vi "CoboltLaser_ComPortClose.vi"(0 "ComPort":refnum<visa-resource-name>, 5 "error in (no error)":errorcluster) -> (19 "error out":errorcluster)   [LabVIEW 2012, in "Cobolt.lvclass"]
uses:
  Template/Cobolt.lvclass
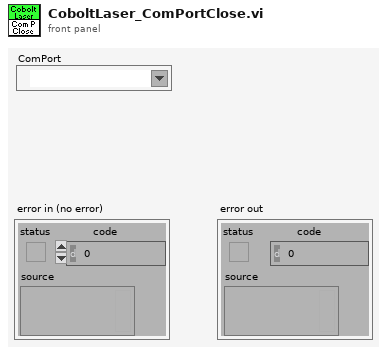
[diagram p1: front panel]
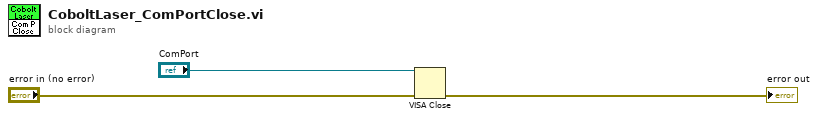
[diagram p0: block diagram]
diagram:
  n1 = VISA Close(VISA resource name="ComPort", error in (no error)="error in (no error)") -> (error out=→"error out":errorcluster)
